vi "Get all Queue References.vi"(8 "error in (no error)":errorcluster, 11 "create if not found? (F)":bool) -> (0 "error out":errorcluster, 1 "Recipes Queue":refnum<queue>, 2 "Saturation Queue":refnum<queue>, 3 "Expansion Queue":refnum<queue>)   [LabVIEW 2017]
uses:
  Recipes/Recipes.lvclass
  Saturation/Saturation.lvclass
  Expansion/Expansion.lvclass
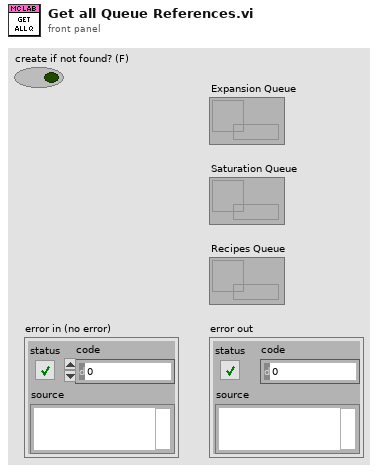
[diagram p1: front panel]
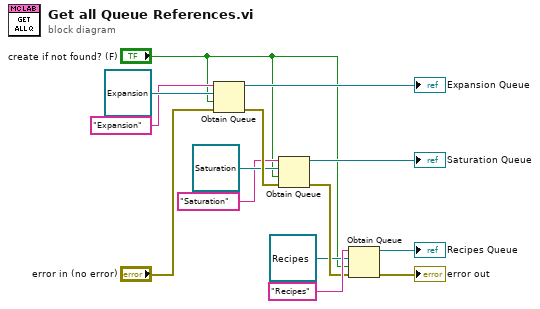
[diagram p0: block diagram]
diagram:
  n1 = Obtain Queue(name (unnamed)="Expansion", element data type=refnum<class "Expansion.lvclass"> refnum, create if not found? (T)="create if not found? (F)", error in (no error)="error in (no error)") -> (queue out=→"Expansion Queue":refnum<queue>, error out=w9:errorcluster)  [unwired: 1 in, 1 out]
  n2 = Obtain Queue(name (unnamed)="Saturation", element data type=refnum<class "Saturation.lvclass"> refnum, create if not found? (T)="create if not found? (F)", error in (no error)=w9) -> (queue out=→"Saturation Queue":refnum<queue>, error out=w12:errorcluster)  [unwired: 1 in, 1 out]
  n3 = Obtain Queue(name (unnamed)="Recipes", element data type=refnum<class "Recipes.lvclass"> refnum ("Recipes.lvclass"), create if not found? (T)="create if not found? (F)", error in (no error)=w12) -> (queue out=→"Recipes Queue":refnum<queue>, error out=→"error out":errorcluster)  [unwired: 1 in, 1 out]
